vi "加减法.vi"() -> ()   [LabVIEW 2014]
panel:
  in  "y 2":dbl
  in  "x 2":dbl
  out "减法":dbl
  out "加法":dbl
  in  "x":dbl
  in  "y":dbl
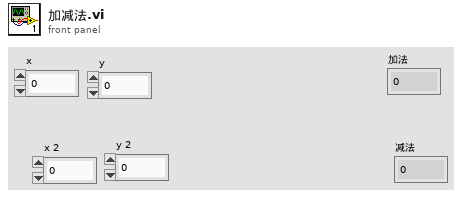
[diagram p1: front panel]
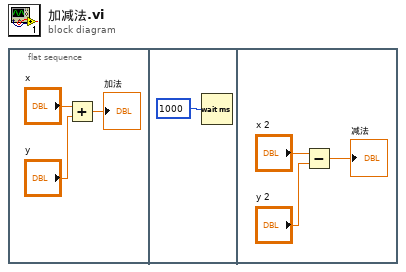
[diagram p0: block diagram]
diagram:
  n1 = flat-sequence {
    frame #0 {
      n2 = Add(x="x", y="y") -> (x+y=→"加法":dbl)
    }
    frame #1 {
      n3 = Wait (ms)(milliseconds to wait=u32 1000 ("等待时间（毫秒）")) -> ()  [unwired: 1 out]
    }
    frame #2 {
      n4 = Subtract(x="x 2", y="y 2") -> (x-y=→"减法":dbl)
    }
  }
